vi "Write RunningAveragePeriodSettings.vi"(8 "error in (no error)":errorcluster, 10 "RunningAveragePeriodSettings":dbl[](array[numeric]), 11 "RunningAverageCalculation in":refnum<class "RunningAverageCalculation.lvclass">) -> (0 "error out":errorcluster, 3 "RunningAverageCalculation out":refnum<class "RunningAverageCalculation.lvclass">)   [LabVIEW 2015, in "RunningAverageCalculation.lvclass"]
uses:
  RunningAverageCalculation.lvclass
  RunningAverageCalculation.lvclass/RunningAverageCalculation.ctl
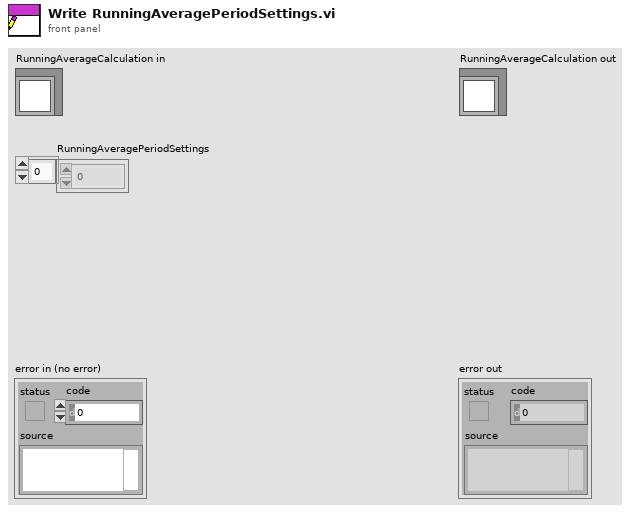
[diagram p1: front panel]
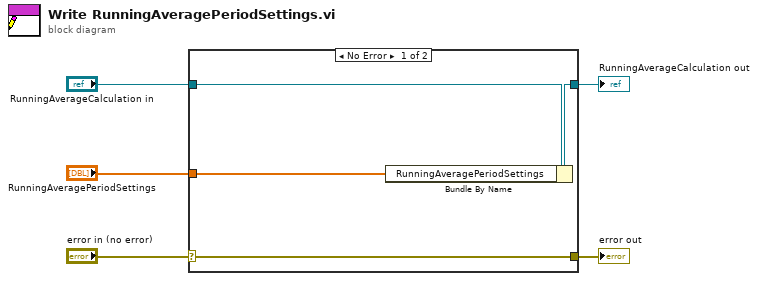
[diagram p0: block diagram]
diagram:
  n1 = case shown="No Error" "error in (no error)" {
    selector: "error in (no error)" -> [w9 w10]
    tunnel: [w9 w10] -> w4
    tunnel: [w7 w11] -> w2
    tunnel: "RunningAverageCalculation in" -> [w8 w11]
    tunnel: "RunningAveragePeriodSettings" -> [w6 _]
    frame No Error {
      n2 = Bundle By Name(cluster=w8, "RunningAveragePeriodSettings"=w6) -> (w7:refnum<class "RunningAverageCalculation.lvclass">)
    }
    frame Error {
    }
  }
  "error out" <- w4
  "RunningAverageCalculation out" <- w2
